vi "FPGA_target_main.vi"() -> ()   [LabVIEW 2014]
doc: "Main VI of the FPGA code. This code implements a pulsed pattern generator on a NI FPGA card, like an PCI-7811R. By this, the timing of an experiment and its experimental procedure can be controlled with a precision down to a few nanoseconds. See the \"blueprints\" in the \"docs\" folder to view the full specifications.\n\nThe main idea is the following. A simple state machine is used to handle the operations states. The data that are uploaded to the FPGA contain commands, pattern data and additional parameters required for some commands. During upload, the data is copied to internal memory of the FPGA. Before the FPGA starts executing commands, the data is copied from the memory to a in internal FIFO. The data in this FIFO is then used during execution of commands in a single-cycle-loop.\n\nmaintainer: Dietrich Beck, d.beck@gsi.de\nauthor: Falk Ziegler\n\nLicense Agreement for this software:\n\nmaintainer: Dietrich Beck, d.beck@gsi.de\nauthor: Falk Ziegler\n\nLicense Agreement for this software:\n\nCopyright (C) 2009\nFalk Ziegler\nInstitut für Physik\nErnst-Moritz-Arndt Universität\nFelix-Hausdorff-Str. 6\n17487 Greifswald\n\nContact: Falk Ziegler, ziegler@physik.uni-greifswald.de\n\nThis program is free software: you can redistribute it and/or modify it under the terms of the GNU General Public License as published by the Free Software Foundation, either version 3 of the License, or (at your option) any later version.\n\nThis program is distributed in the hope that it will be useful, but WITHOUT ANY WARRANTY; without even the implied warranty of MERCHANTABILITY or FITNESS FOR A PARTICULAR PURPOSE. See the GNU General Public License for more details.\n\nYou should have received a copy of the GNU General Public License along with this program. If not, see <http://www.gnu.org/licenses/>.\n\nFor all questions and ideas contact: ziegler@physik.uni-greifswald.de or d.beck@gsi.de\nLast update: 01-Sep-2009"
uses:
  <vilib>/eio/EIONode/EIONode.xnode
  FPGA_target_state_type.ctl
  <vilib>/rvi/DataTransferAndStorage/Container/XNode/niFpgaContainer.xnode
  <vilib>/Platform/TimedLoop/XDataNode/XDataNode.xnode
  <vilib>/Platform/TimedLoop/XDataNode/nitl_modes.ctl
  <vilib>/Platform/TimedLoop/XDataNode/XDNodeRunTimeDep.lvlib
  <vilib>/Platform/TimedLoop/XDataNode/wakeup.ctl
  <vilib>/Platform/TimedLoop/XDataNode/timing_clust.ctl
  <vilib>/rvi/eio/common/nirviEmuTemplateMethod_errors.vi
  <vilib>/rvi/interface/RandomDataEmulation/nirviRandomDataFpgaReadWriteTemplate.vi
  <vilib>/rvi/Memory/Memory_Emulation/nirvimemoryEmulation.vi
  <vilib>/rvi/Memory/Memory_Emulation/nirvimemoryFastEmulation.vi
panel:
  in  "useJump":bool
  out "ticks_per_us":i32
  out "revision":i32
  in  "query":bool
  out "elements_loaded":i32
  in  "replace":bool
  in  "run":bool
  in  "load":bool
  in  "reset":bool
  in  "mem_addr":u32
  out "error_code":u8
  out "state":T1
  out "number_of_cmds":u32
  out "stop_addr":u32
  in  "stop":bool
  out "start_sctl":bool
  out "fifo_empty":bool
  in  "continuous":bool
  out "stop_sctl":bool
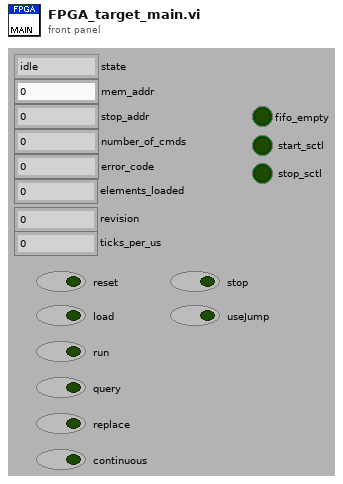
[diagram p1: front panel]
types:
  T1 = typedef "NI-FPGA_PPG_Driver.lvlib/FPGA_target_state_type.ctl" = enum16{"idle", "reset", "query", "load", "run", "stopped"}
  T2 = cluster{"mem_addr":u32, "cmd":u8, "cmd_data":u32}
  T3 = typedef "XDNodeRunTimeDep.lvlib/timing_clust.ctl" = cluster{"Expected End [f-1]":u64, "Actual End [f-1]":u64, "Finished Late? [f-1]":bool, "Expected End [i-1]":u64, "Actual End [i-1]":u64, "Finished Late? [i-1]":bool, "Expected Start [i]":u64, "Actual Start [i]":u64, "Expected Start [f]":u64, "Actual Start [f]":u64, "Source Name":string, "Structure Name":string, "Period":i64, "Deadline":i64, "Offset":i64, "Start":i64, "Priority":i32, "Timeout":i32, "Mode":T4, "Wakeup Reason":T5, "Error":errorcluster, "Source Type":string, "Secondary Source Type":string, "Global End Time":u64, "Global Start Time":u64, "Frame Duration":u64, "Iteration Duration":u64, "Assigned CPU":i32, "I/O Scan Engine Mode":u32}
  T4 = typedef "XDNodeRunTimeDep.lvlib/nitl_modes.ctl" = enum32{"No Change", "Process missed periods, maintain original phase", "Discard missed periods, maintain original phase", "Process missed periods, ignore original phase", "Discard missed periods, ignore original phase"}
  T5 = typedef "XDNodeRunTimeDep.lvlib/wakeup.ctl" = enum32{"Normal", "Aborted", "Asynchronous wakeup", "Timing source error", "Timed loop error", "Timeout"}
  T6 = typedef "FPGA_32BitPattern_data_type.ctl" = cluster{"port0":u8, "port1":u8}
  T7 = typedef "FPGA_cmd_data_type.ctl" = cluster{"mem_addr":u32, "cmd":u8, "cmd_data":u32}
  T8 = typedef "FPGA_mem_data_type.ctl" = cluster{"mem_addr":u32, "cmd":u8, "cmd_data":u32, "C1":u16}
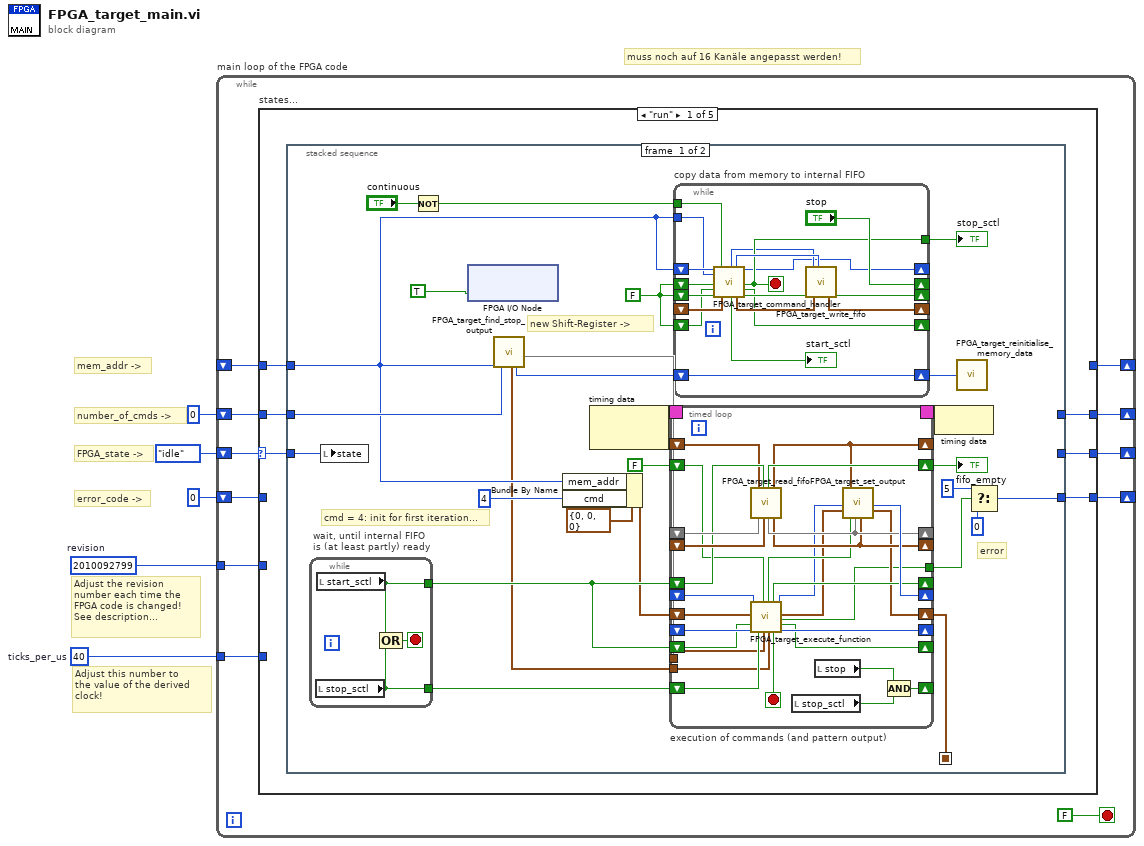
[diagram p0: block diagram]
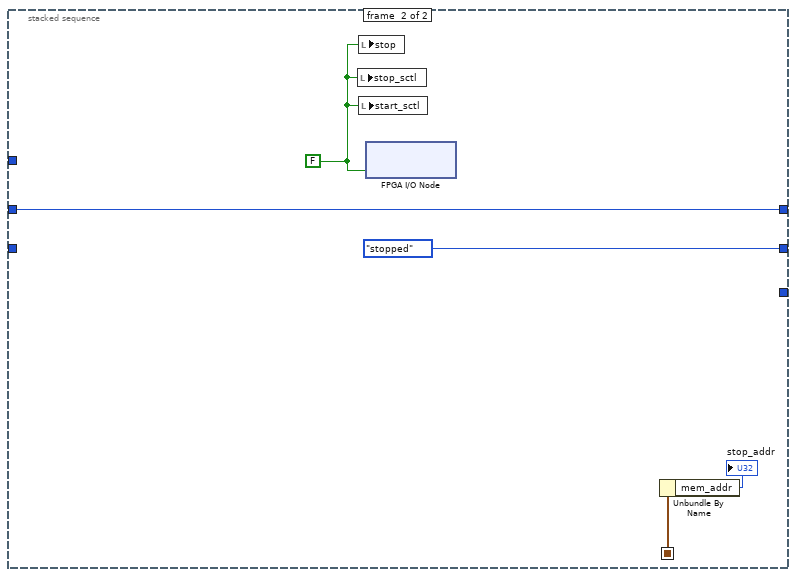
[diagram p2: hidden frame]
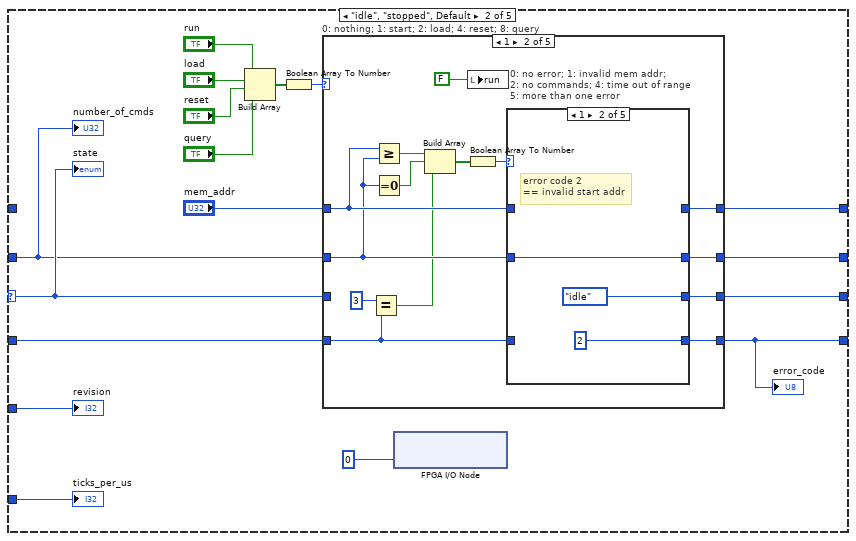
[diagram p3: hidden frame]
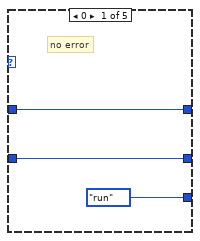
[diagram p5: hidden frame]
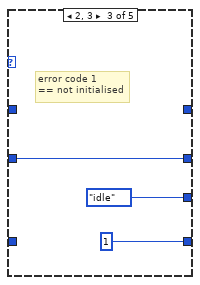
[diagram p6: hidden frame]
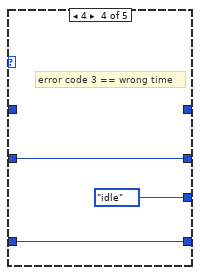
[diagram p7: hidden frame]
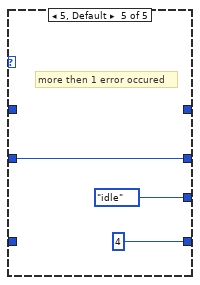
[diagram p8: hidden frame]
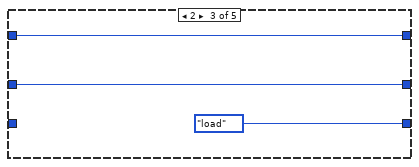
[diagram p9: hidden frame]
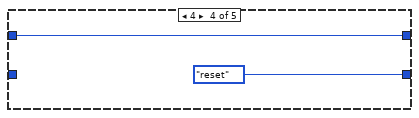
[diagram p10: hidden frame]
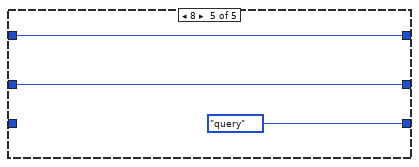
[diagram p11: hidden frame]
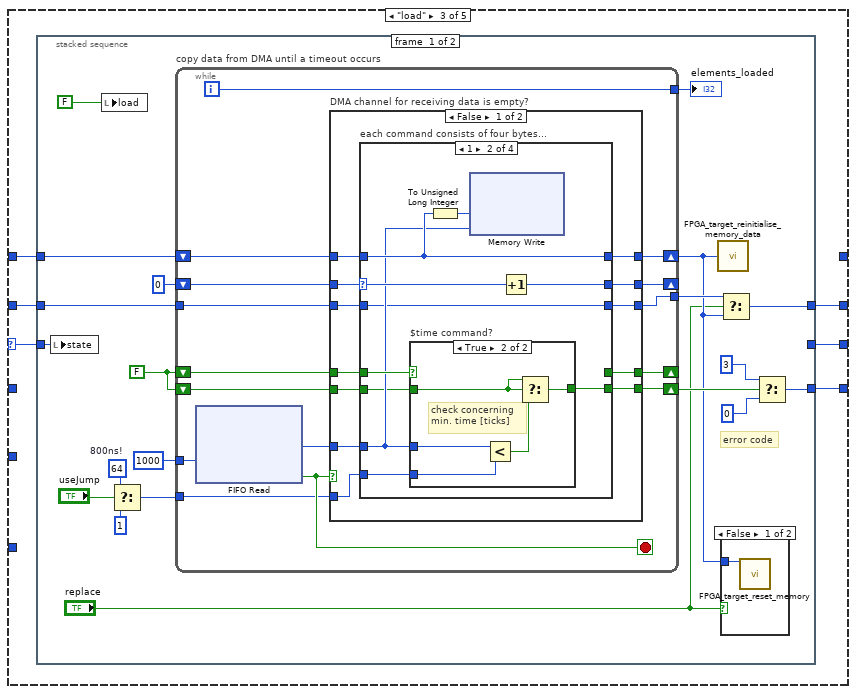
[diagram p12: hidden frame]
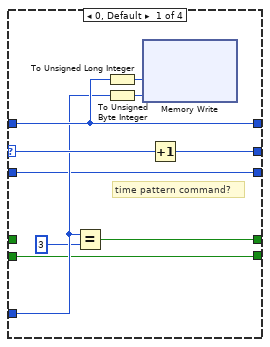
[diagram p14: hidden frame]
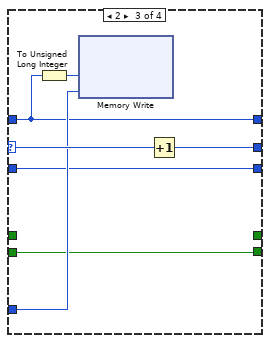
[diagram p16: hidden frame]
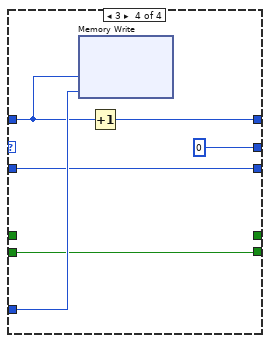
[diagram p17: hidden frame]
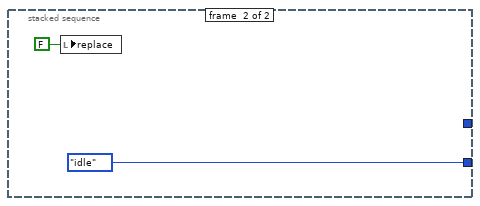
[diagram p19: hidden frame]
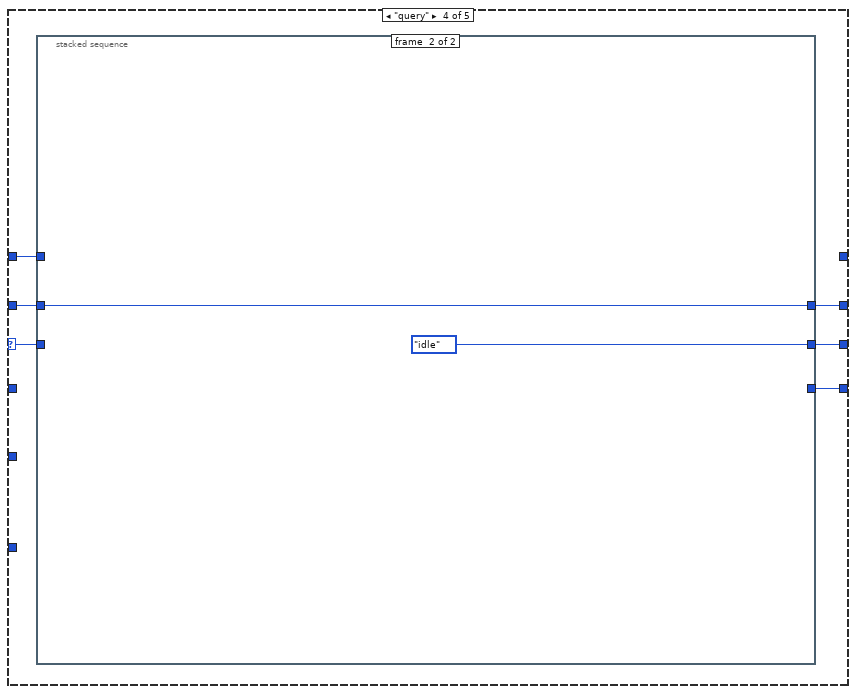
[diagram p20: hidden frame]
diagram:
  w1 = 40  # ticks_per_us
  w2 = 2010092799  # revision
  # "muss noch auf 16 Kanäle angepasst werden!"
  # "Adjust this number to\nthe value of the derived\nclock!"
  # "Adjust the revision\nnumber each time the\nFPGA code is changed!\nSee description..."
  # "error_code ->"
  # "FPGA_state ->"
  # "number_of_cmds ->"
  # "mem_addr ->"
  n1 = while "main loop of the FPGA code" {
    shift-right: [w14] -> _
    shift-left: FPGA_target_state_type."idle" ("State") -> [w16]
    shift-right: [w13] -> _
    shift-left: _ -> [w12]
    shift-right: [w11] -> _
    shift-left: u8 0 -> [w10]
    shift-right: [w9] -> _
    shift-left: u32 0 ("mem_addr") -> [w8]
    tunnel: w2 -> [w7]
    tunnel: w1 -> [w6]
    stop <- FALSE stop-if-true
    n2 = case "states..." shown="\"run\"" w16 {
      selector: w16 -> [w21 w125 w170 w268 w309]
      tunnel: [w20 w124 w169 w267 FPGA_target_state_type."idle" ("State")] -> w14
      tunnel: [_ w123 _ _ _] -> w13
      tunnel: w12 -> [w22 _ w171 w269 _]
      tunnel: [w17 w111 w167 w265 _] -> w11
      tunnel: w10 -> [_ w122 _ _ _]
      tunnel: [w19 w120 w168 w266 _] -> w9
      tunnel: w8 -> [w18 w121 w166 w264 _]
      tunnel: w7 -> [_ w110 _ _ _]
      tunnel: w6 -> [_ w109 _ _ _]
      frame "run" {
        n3 = stacked-sequence {
          seq-local: [w47 _] -> [_ w106]
          tunnel: w22 -> [w28 _]
          tunnel: w21 -> [w32 _]
          tunnel: [_ FPGA_target_state_type."stopped" ("State")] -> w20
          tunnel: [_ w107] -> w19
          tunnel: w18 -> [w48 w107]
          tunnel: [w46 _] -> w17
          frame #0 {
            w25 = FALSE ("DO_is_active")
            # "cmd = 4: init for first iteration..."
            # "new Shift-Register ->"
            # "error"
            n4 = while "wait, until internal FIFO\nis (at least partly) ready" {
              tunnel: [w102] -> w45
              tunnel: [w101] -> w42
              stop <- w103 stop-if-true
              n5 = local read "stop_sctl"() -> (w102:bool)
              n6 = local read "start_sctl"() -> (w101:bool)
              n7 = Compound Arithmetic op=OR(w101, w102) -> (w103:bool)
            }
            n8 = local write "state"(w32) -> ()
            n9 = Not(x="continuous") -> (.not. x?=w38:bool)
            n10 = xnode "FPGA I/O Node"("DO_state"=TRUE ("DO_is_active")) -> ()  [unwired: 1 in, 1 out]
            n11 = call "FPGA_target_find_stop_output.vi"("start_addr"=w28, "number_cmds_in"=w48) -> (9:w26, "C1_data"=w27:T6, "number_cmds_dup"=w39:u32)  [unwired: 14 in, 1 out]
            n12 = Bundle By Name(cluster=T2 {"mem_addr"=0, "cmd"=0, "cmd_data"=0} ("data_out"), "mem_addr"=w28, "cmd"=u8 4) -> (w36:T2)
            n13 = node-c288() -> (w24:T3)  [unwired: 1 in]
            n14 = timed-loop "execution of commands (and pattern output)" {
              shift-right: [w58] -> _
              shift-left: _ -> [w57]
              shift-right: [w74] -> _
              shift-left: _ -> [w77]
              shift-right: [w73] -> _
              shift-left: _ -> [w76]
              shift-right: [w75] -> _
              shift-left: _ -> [w66]
              shift-right: [w70] -> _
              shift-left: w42 -> [w67]
              shift-right: [w49] -> _
              shift-left: w45 -> [w72]
              shift-right: [w69] -> w44
              shift-left: FALSE ("fifo_empty") -> [w53]
              shift-right: [w55] -> w47
              shift-left: w36 -> [w54]
              shift-right: [w64] -> _
              shift-left: _ -> [w63]
              tunnel: w26 -> [w62]
              tunnel: w27 -> [w61]
              shift-right: [w59] -> _
              shift-left: w42 -> [w60]
              tunnel: [w52] -> w35
              timing: w24 -> [_]
              timing-out: [_] -> w23
              stop <- w68 stop-if-true
              n15 = call "FPGA_target_read_fifo.vi"("data_in"=w57, 7:w77, "read_fifo"=w67, "C1_in"=w76) -> ("fifo_empty"=w69:bool, 11:w74, "data_out"=w58:T7, "C1_out"=w73:T6)  [unwired: 12 in]
              n16 = call "FPGA_target_execute_function.vi"("tick_count_in"=w66, "data_in"=w54, "set_stop_output_in"=w60, "input_data_in"=w63, "stop_request"=w72, "fifo_empty_in"=w53, 9:w62, "C1_data"=w61) -> ("set_output"=w71:bool, "read_fifo"=w70:bool, "stop"=w68:bool, "tick_count_out"=w65:u32, "data_dup"=w56:T7, "fifo_empty_out"=w52:bool, "set_stop_output_out"=w59:bool, "input_data_out"=w64:u8)  [unwired: 4 in]
              n17 = local read "stop_sctl"() -> (w51:bool)
              n18 = local read "stop"() -> (w50:bool)
              n19 = call "FPGA_target_set_output.vi"("tick_count_in"=w65, "data_in"=w56, "new_data_in"=w58, "set_outputs"=w71, 9:w74, "C1_data"=w73) -> ("tick_count_out"=w75:u32, "data_out"=w55:T7)  [unwired: 12 in]
              n20 = Compound Arithmetic op=AND(w50, w51) -> (w49:bool)
            }
            "fifo_empty" <- w44
            n21 = while "copy data from memory to internal FIFO" {
              shift-right: [w91] -> _
              shift-left: _ -> [w90]
              tunnel: w28 -> [w85]
              tunnel: w38 -> [w87]
              shift-right: [w100] -> w41
              shift-left: w39 -> [w100]
              shift-right: [w89] -> _
              shift-left: w25 -> [w98]
              shift-right: ["stop"] -> _
              shift-left: w25 -> [w93]
              shift-right: [w84] -> _
              shift-left: w28 -> [w94]
              tunnel: [w88] -> w31
              shift-right: [w82] -> _
              shift-left: w25 -> [w83]
              stop <- w88 stop-if-true
              n22 = call "FPGA_target_command_handler.vi"("mem_addr_in"=w94, "mem_addr_start"=w85, "force_stop"=w93, "stop_execution_in"=w83, "FIFO_full"=w98, "continuous"=w87, "mem_data_in"=w90) -> ("mem2_addr"=w86:u32, "start_sctl"=→"start_sctl":bool, "mem2_data"=w95:u16, "mem_data_out"=w92:T8, "mem_addr_ out"=w84:u32, "stop_execution_out"=w88:bool, "stop_triggered"=w82:bool, "write_FIFO"=w99:bool)  [unwired: 5 in]
              n23 = call "FPGA_target_write_fifo.vi"("write_FIFO"=w99, "mem2_addr_in"=w86, "mem_data_in"=w92, "mem2_data"=w95) -> ("mem_data_dup"=w91:T8, "FIFO_full"=w89:bool)  [unwired: 13 in, 1 out]
            }
            "stop_sctl" <- w31
            n24 = node-c288(w23) -> ()
            n25 = call "FPGA_target_reinitialise_memory_data.vi"("number_cmds"=w41) -> ()
            n26 = Select(t=u8 5, s=w35, f=u8 0) -> (s? t:f=w46:u8)
          }
          frame #1 {
            w104 = FALSE ("DO_is_active")
            n27 = local write "stop_sctl"(w104) -> ()
            n28 = local write "stop"(w104) -> ()
            n29 = local write "start_sctl"(w104) -> ()
            n30 = xnode "FPGA I/O Node"("DO_state"=w104) -> ()  [unwired: 1 in, 1 out]
            n31 = Unbundle By Name(w106) -> ("mem_addr"=→"stop_addr":u32)
          }
        }
      }
      frame "idle", "stopped", Default {
        n32 = Build Array("run", "load", "reset", "query") -> (w115:bool[])
        n33 = Boolean Array To Number(Boolean array=w115) -> (number=w116:u8)
        n34 = case "0: nothing; 1: start; 2: load; 4: reset; 8: query" shown="1" w116 {
          tunnel: [w128 w142 FPGA_target_state_type."load" ("state") FPGA_target_state_type."reset" ("state") FPGA_target_state_type."query" ("state")] -> w124
          tunnel: [_ w136 w159 _ w163] -> w123
          tunnel: "mem_addr" -> [_ w137 w159 _ w163]
          tunnel: w125 -> [w128 _ _ _ _]
          tunnel: [w127 w133 _ _ _] -> w111
          tunnel: w122 -> [w127 w130 _ _ _]
          tunnel: w121 -> [w126 w135 w158 w161 w164]
          tunnel: [w126 w134 w158 w161 w164] -> w120
          frame 0, Default {
          }
          frame 1 {
            n35 = Equal?(x=u8 3 ("y"), y=w130) -> (x = y?=w132:bool)
            n36 = Greater Or Equal?(x=w137, y=w135) -> (x >= y?=w141:bool)
            n37 = Equal To 0?(x=w135) -> (x = 0?=w140:bool)
            n38 = Build Array(w141, w140, w132) -> (w139:bool[])
            n39 = local write "run"(FALSE) -> ()
            n40 = Boolean Array To Number(Boolean array=w139) -> (number=w138:u8)
            n41 = case "0: no error; 1: invalid mem addr; \n2: no commands; 4: time out of range\n5: more than one error" shown="1" w138 {
              tunnel: [FPGA_target_state_type."run" ("state") FPGA_target_state_type."idle" ("state") FPGA_target_state_type."idle" ("state") FPGA_target_state_type."idle" ("state") FPGA_target_state_type."idle" ("state")] -> w142
              tunnel: w137 -> [w144 _ _ _ _]
              tunnel: [w144 _ _ _ _] -> w136
              tunnel: w135 -> [w143 w147 w150 w154 w157]
              tunnel: [w143 w147 w150 w154 w157] -> w134
              tunnel: [_ u8 2 u8 1 w152 u8 4 ("f")] -> w133
              tunnel: w130 -> [_ _ _ w152 _]
              frame 0 {
                # "no error"
              }
              frame 1 {
                # "error code 2 \n== invalid start addr"
              }
              frame 2, 3 {
                # "error code 1 \n== not initialised"
              }
              frame 4 {
                # "error code 3 == wrong time"
              }
              frame 5, Default {
                # "more then 1 error occured"
              }
            }
          }
          frame 2 {
          }
          frame 4 {
          }
          frame 8 {
          }
        }
        "error_code" <- w111
        n42 = xnode "FPGA I/O Node"("TriggerIn_0-7"=u8 0 ("DI_port0")) -> ()  [unwired: 1 in, 1 out]
        "state" <- w125
        "number_of_cmds" <- w121
        "revision" <- w110
        "ticks_per_us" <- w109
      }
      frame "load" {
        n43 = stacked-sequence {
          tunnel: w171 -> [w177 _]
          tunnel: w170 -> [w190 _]
          tunnel: [_ FPGA_target_state_type."idle" ("State")] -> w169
          tunnel: [w181 _] -> w168
          tunnel: [w184 _] -> w167
          tunnel: w166 -> [w183 _]
          frame #0 {
            w172 = u32 64  # 800ns!
            w188 = FALSE
            # "error code"
            n44 = local write "state"(w190) -> ()
            n45 = local write "load"(FALSE ("load")) -> ()
            n46 = Select(t=w172, s="useJump", f=u32 1 ("x")) -> (s? t:f=w173:u32)
            n47 = while "copy data from DMA until a timeout occurs" {
              tunnel: 1000 -> [w202]
              shift-right: [w203] -> _
              shift-left: u16 0 -> [w206]
              shift-right: [w204] -> w180
              shift-left: w177 -> [w205]
              shift-right: [w199] -> _
              shift-left: w188 -> [w200]
              shift-right: [w197] -> w187
              shift-left: w188 -> [w198]
              tunnel: w183 -> [w196]
              tunnel: [w195] -> w182
              tunnel: [w194] -> w176
              tunnel: w173 -> [w193]
              i -> [w194]
              stop <- w201 stop-if-true
              n48 = xnode ("FIFO Read")("Timeout"=w202) -> ("Element"=w207:u32, "Timed Out?"=w201:bool)  [unwired: 1 in, 1 out]
              n49 = case "DMA channel for receiving data is empty?" shown="False" w201 {
                tunnel: w207 -> [w218 _]
                tunnel: w206 -> [w219 _]
                tunnel: w205 -> [w217 w261]
                tunnel: [w215 w261] -> w204
                tunnel: [w216 _] -> w203
                tunnel: w200 -> [w214 _]
                tunnel: [w213 _] -> w199
                tunnel: w198 -> [w212 w260]
                tunnel: [w211 w260] -> w197
                tunnel: w196 -> [w210 w259]
                tunnel: [w209 w259] -> w195
                tunnel: w193 -> [w208 _]
                frame False {
                  n50 = case "each command consists of four bytes..." shown="1" w219 {
                    selector: w219 -> [w229 w239 w252 _]
                    tunnel: w218 -> [w223 w234 w250 w256]
                    tunnel: w217 -> [w226 w236 w248 w255]
                    tunnel: [w226 w236 w248 w257] -> w215
                    tunnel: [w228 w238 w251 u16 0] -> w216
                    tunnel: w214 -> [_ w235 _ _]
                    tunnel: [w224 _ _ _] -> w213
                    tunnel: w212 -> [w221 w233 w247 w254]
                    tunnel: [w221 w232 w247 w254] -> w211
                    tunnel: w210 -> [w220 w231 w246 w253]
                    tunnel: [w220 w231 w246 w253] -> w209
                    tunnel: w208 -> [_ w230 _ _]
                    frame 0, Default {
                      # "time pattern command?"
                      n51 = Equal?(x=w223, y=u32 3 ("x")) -> (x = y?=w224:bool)
                      n52 = To Unsigned Long Integer(number=w226) -> (unsigned 32bit integer=w227:u32)
                      n53 = To Unsigned Byte Integer(number=w223) -> (unsigned 8bit integer=w225:u8)
                      n54 = xnode ("Memory Write")("Address"=w227, "Data"=w225) -> ()  [unwired: 1 in, 1 out]
                      n55 = Increment(x=w229) -> (x+1=w228:u16)
                    }
                    frame 1 {
                      n56 = case "$time command?" shown="True" w235 {
                        tunnel: w234 -> [_ w244]
                        tunnel: w233 -> [w240 w245]
                        tunnel: [w240 w242] -> w232
                        tunnel: w230 -> [_ w241]
                        frame False {
                        }
                        frame True {
                          # "check concerning\nmin. time [ticks]"
                          n57 = Less?(x=w244, y=w241) -> (x < y?=w243:bool)
                          n58 = Select(t=w245, s=w245, f=w243) -> (s? t:f=w242:bool)
                        }
                      }
                      n59 = To Unsigned Long Integer(number=w236) -> (unsigned 32bit integer=w237:u32)
                      n60 = xnode ("Memory Write")("Address"=w237, "Data"=w234) -> ()  [unwired: 1 in, 1 out]
                      n61 = Increment(x=w239) -> (x+1=w238:u16)
                    }
                    frame 2 {
                      n62 = To Unsigned Long Integer(number=w248) -> (unsigned 32bit integer=w249:u32)
                      n63 = xnode ("Memory Write")("Address"=w249, "Data"=w250) -> ()  [unwired: 1 in, 1 out]
                      n64 = Increment(x=w252) -> (x+1=w251:u16)
                    }
                    frame 3 {
                      n65 = xnode ("Memory Write")("Address"=w255, "Data"=w256) -> ()  [unwired: 1 in, 1 out]
                      n66 = Increment(x=w255) -> (x+1=w257:u32)
                    }
                  }
                }
                frame True {
                }
              }
            }
            "elements_loaded" <- w176
            n67 = call "FPGA_target_reinitialise_memory_data.vi"("number_cmds"=w180) -> ()
            n68 = Select(t=w182, s="replace", f=w180) -> (s? t:f=w181:u32)
            n69 = case shown="False" "replace" {
              tunnel: w180 -> [w192 _]
              frame False {
                n70 = call "FPGA_target_reset_memory.vi"("mem_addr_in"=w192) -> ()  [unwired: 18 in, 1 out]
              }
              frame True {
              }
            }
            n71 = Select(t=u8 3, s=w187, f=u8 0) -> (s? t:f=w184:u8)
          }
          frame #1 {
            n72 = local write "replace"(FALSE ("replace")) -> ()
          }
        }
      }
      frame "query" {
        n73 = stacked-sequence {
          tunnel: w269 -> [w280 _]
          tunnel: w268 -> [_ _]
          tunnel: [_ FPGA_target_state_type."idle" ("State")] -> w267
          tunnel: [_ w304] -> w266
          tunnel: [w270 _] -> w265
          tunnel: w264 -> [_ w304]
          frame #0 {
            # "error"
            n74 = local write "query"(FALSE ("load")) -> ()
            n75 = call "FPGA_target_read_memory.vi"("addr_in"=w280) -> ("data_mem0"=w279:u8, 9:w277, "data_mem2"=w276:u16, "data_mem3"=w278:u32, "addr_dup"=w275:u32)  [unwired: 13 in, 1 out]
            n76 = while "for all bytes of a command" {
              tunnel: w279 -> [w290]
              tunnel: w278 -> [w289]
              tunnel: w277 -> [w288]
              tunnel: w276 -> [w287]
              tunnel: w275 -> [_]
              tunnel: 3 -> [w285]
              tunnel: [w282] -> w273
              i -> [w286]
              stop <- w283 stop-if-true
              n77 = Equal?(x=w286, y=w285) -> (x = y?=w284:bool)
              n78 = case "each command has four bytes..." shown="0, Default" w286 {
                tunnel: w290 -> [w294 _ _ _]
                tunnel: [w291 w296 w299 w302] -> w282
                tunnel: w289 -> [_ w295 _ _]
                tunnel: w288 -> [_ _ w298 _]
                tunnel: w287 -> [_ _ _ w301]
                frame 0, Default {
                  n79 = To Unsigned Long Integer(number=w294) -> (unsigned 32bit integer=w293:u32)
                  n80 = xnode ("FIFO Write")("Element"=w293, "Timeout"=0) -> ("Timed Out?"=w291:bool)  [unwired: 1 in, 1 out]
                }
                frame 1 {
                  n81 = xnode ("FIFO Write")("Element"=w295, "Timeout"=0) -> ("Timed Out?"=w296:bool)  [unwired: 1 in, 1 out]
                }
                frame 2 {
                  n82 = xnode ("FIFO Write")("Element"=w298, "Timeout"=0) -> ("Timed Out?"=w299:bool)  [unwired: 1 in, 1 out]
                }
                frame 3 {
                  n83 = xnode ("FIFO Write")("Element"=w301, "Timeout"=0) -> ("Timed Out?"=w302:bool)  [unwired: 1 in, 1 out]
                }
              }
              n84 = Compound Arithmetic op=OR(w282, w284) -> (w283:bool)
            }
            n85 = Select(t=u8 6, s=w273, f=u8 0) -> (s? t:f=w270:u8)
          }
          frame #1 {
          }
        }
      }
      frame "reset" {
        w306 = FALSE ("reset")
        n86 = local write "continuous"(w306) -> ()
        n87 = local write "reset"(w306) -> ()
        n88 = local write "state"(w309) -> ()
        n89 = call "FPGA_target_reset_memory.vi"("mem_addr_in"=u32 0) -> ()  [unwired: 18 in, 1 out]
      }
    }
  }
